vi "iconPixmap.vi"(8 "Error In":errorcluster, 11 "QMessageBox In":refnum<class "QMessageBox.lvclass">) -> (0 "Error Out":errorcluster, 2 "Value":refnum<class "QPixmap.lvclass">, 3 "QMessageBox Out":refnum<class "QMessageBox.lvclass">)   [LabVIEW 2014, in "QMessageBox.lvclass"]
doc: "LabVIEW-specific documentation is not yet available. See <b>http://doc.qt.io/qt-5/QMessageBox.html#iconPixmap</b>"
uses:
  QMessageBox.lvclass
  Qt GUI/QPixmap/QPixmap.lvclass
  LQ Core/LQIdentity/LQIdentity.lvclass/LQIdentity.ctl
  LQ Core/LQSerialData/LQSerialData.lvclass/LQSerialData.ctl
  LQ Core/LQ Core.lvlib
  LQ Core/LQIdentity/LQIdentity.lvclass
  LQ Core/LQSerialData/LQSerialData.lvclass
panel:
  # "Copyright (c) 2016 Sze Howe Koh\n\nThis Source Code Form is subject to the terms of the Mozilla Public\nLicense, v. 2.0. If a copy of the MPL was not distributed with this\nfile, You can obtain one at http://mozilla.org/MPL/2.0/."
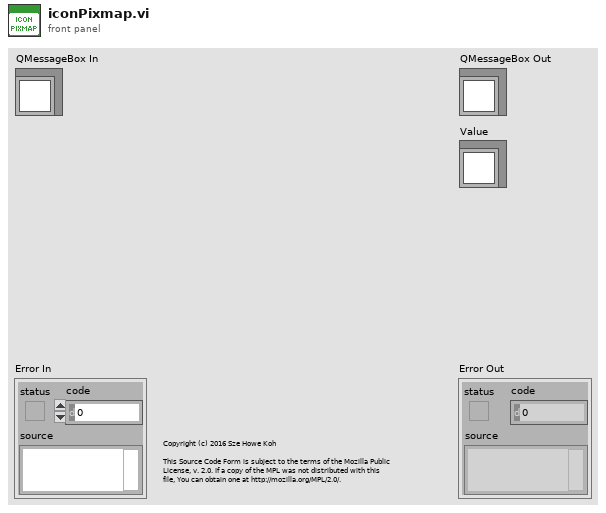
[diagram p1: front panel]
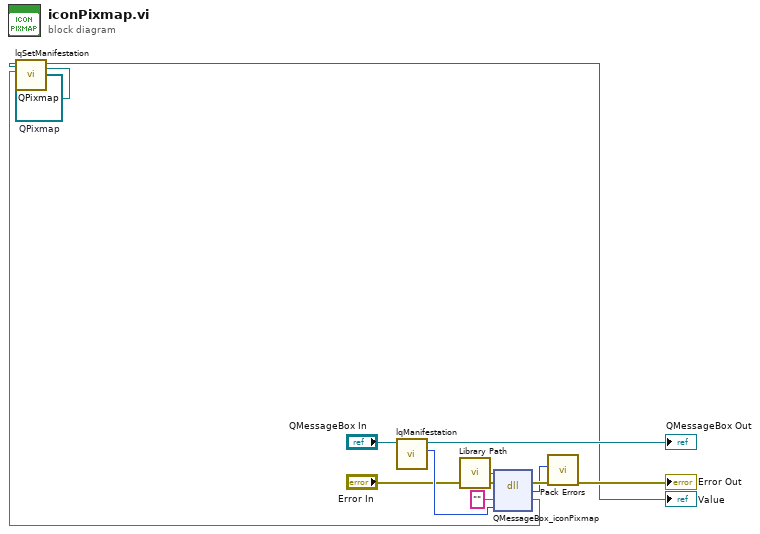
[diagram p0: block diagram]
diagram:
  w1 = refnum<class "QPixmap.lvclass"> refnum  # QPixmap
  n1 = call "lqManifestation.vi"("LQIdentity in"="QMessageBox In") -> ("Manifestation"=w8:u64, "LQIdentity out"=→"QMessageBox Out":refnum<class "QMessageBox.lvclass">)  [unwired: 9 in]
  n2 = call "Library Path.vi"() -> ("Library Path"=w9:path)
  n3 = dll-call lib="?" fn="QMessageBox_iconPixmap"(path in=w9, error in="Error In", "_retVal"="" ("retVal"), "_instance"=w8) -> (error out=w6:errorcluster, w4:i32, "_retVal"=w2:string)  [unwired: 2 in, 1 out]
  n4 = call "lqSetManifestation.vi"("Manifestation"=w2, "LQSerialData in"=w1) -> ("LQSerialData out"=→"Value":refnum<class "QPixmap.lvclass">)  [unwired: 8 in, 1 out]
  n5 = call "Pack Errors.vi"("Error In"=w6, "Error Code"=w4) -> ("Error Out"=→"Error Out":errorcluster)  [unwired: 9 in]
